vi "Version_4.9_8_on-chip_valves_for25ulSyringe_withModfied_Plunging.vi"() -> ()   [LabVIEW 2020] (continued)
                                n5068 = call "ProcessCompletionWaiter (SubVI).vi"("VISA Refnum in"=w5469) -> ()  [unwired: 11 in]
                                }
                                frame #2 {
                                # "Switch to Port-10"
                                # "Port-10 of the pump is conncted to column-2 of chip"
                                n5069 = local read "VISA Refnum in\nfor Pump"() -> (w5472:refnum<visa-resource-name>)
                                n5070 = call "PortChanger (SubVI).vi"("Port Number"="10", "VISA Refnum in"=w5472) -> ()  [unwired: 10 in]
                                }
                                frame #3 {
                                n5071 = local read "Stopper that ends \nthe main loops"() -> (w5473:bool)
                                n5072 = local read "VISA Refnum in\nfor Pump"() -> (w5474:refnum<visa-resource-name>)
                                n5073 = case shown="True" w5473 {
                                frame False {
                                }
                                frame True {
                                n5074 = local read "VISA Refnum in\nfor Pump"() -> (w5475:refnum<visa-resource-name>)
                                n5075 = call "HardStopCurrentProcess (SubVI).vi"("VISA Refnum in"=w5475) -> ()  [unwired: 11 in]
                                }
                                }
                                n5076 = call "ProcessCompletionWaiter (SubVI).vi"("VISA Refnum in"=w5474) -> ()  [unwired: 11 in]
                                }
                                frame #4 {
                                # "Keeps the AMF valve after column-1 open and valve after column-2 closed"
                                n5077 = local read "Buffer-A2 Pumping\nResolution"() -> (w5487:T2)
                                n5078 = local read "VISA Refnum in\nfor Pump"() -> (w5489:refnum<visa-resource-name>)
                                n5079 = local read "f"() -> (w5481:dbl)
                                n5080 = local write "Valve V3 Open"(TRUE ("Valve V3 Open")) -> ()
                                n5081 = local write "Valve V2 Open"(FALSE ("Valve V2 Open")) -> ()
                                n5082 = local write "Valve V4 Open"(TRUE ("Valve V4 Open")) -> ()
                                n5083 = local write "Valve V1 Open"(FALSE ("Valve V1 Open")) -> ()
                                n5084 = local read "Volume of Syringe"() -> (w5488:dbl)
                                n5085 = call "GoToAbsolutePosition(SubVI).vi"("Absolute Volume Position in Syringe (in ul)"=0.0 ("Volume to be Dispensed"), "Volume of Syringe"=w5488, "Resolution of Pumping"=w5487, "Flow Rate (ul/min)"=w5481, "VISA Refnum in"=w5489) -> ()  [unwired: 6 in, 1 out]
                                n5086 = local write "External Valve \nOpen"(FALSE ("External Valve \nOpen")) -> ()
                                n5087 = local write "Valve V8 Open"(FALSE ("Valve V8 Open")) -> ()
                                n5088 = local write "Valve V5 Open"(TRUE ("Valve V5 Open")) -> ()
                                n5089 = local write "Valve V6 Open"(FALSE ("Valve V6 Open")) -> ()
                                n5090 = local write "Valve V7 Open"(TRUE ("Valve V7 Open")) -> ()
                                }
                                frame #5 {
                                n5091 = local read "VISA Refnum in\nfor Pump"() -> (w5490:refnum<visa-resource-name>)
                                n5092 = call "ProcessCompletionWaiter (SubVI).vi"("VISA Refnum in"=w5490) -> ()  [unwired: 11 in]
                                }
                                frame #6 {
                                # "Change the port back to Buffer-C1"
                                n5093 = local read "VISA Refnum in\nfor Pump"() -> (w5492:refnum<visa-resource-name>)
                                n5094 = local read "Port for \nC1-Equilibriation"() -> (w5491:string)
                                n5095 = call "PortChanger (SubVI).vi"("Port Number"=w5491, "VISA Refnum in"=w5492) -> ()  [unwired: 10 in]
                                }
                                frame #7 {
                                n5096 = local read "VISA Refnum in\nfor Pump"() -> (w5493:refnum<visa-resource-name>)
                                n5097 = call "ProcessCompletionWaiter (SubVI).vi"("VISA Refnum in"=w5493) -> ()  [unwired: 11 in]
                                }
                              }
                            }
                            n5098 = local write "Reminder of the \nVolume to be \nPumped"(w5460) -> ()
                          }
                          frame #5 {
                            # "Washes the SEC column"
                            n5099 = stacked-sequence {
                              frame #0 {
                                n5100 = local read "Buffer-A2 Pumping\nResolution"() -> (w5496:T2)
                                n5101 = local read "VISA Refnum in\nfor Pump"() -> (w5498:refnum<visa-resource-name>)
                                n5102 = local read "Reminder of the \nVolume to be \nPumped"() -> (w5494:dbl)
                                n5103 = local read "Volume of Syringe"() -> (w5497:dbl)
                                n5104 = call "RPickUp(SubVI).vi"("Volume to be picked up"=w5494, "Volume of Syringe"=w5497, "Resolution of PickUP"=w5496, "PickUp Flow Rate (ul/min)"=150.0, "VISA Refnum in"=w5498) -> ()  [unwired: 6 in, 1 out]
                              }
                              frame #1 {
                                n5105 = local read "Stopper that ends \nthe main loops"() -> (w5499:bool)
                                n5106 = local read "VISA Refnum in\nfor Pump"() -> (w5500:refnum<visa-resource-name>)
                                n5107 = case shown="True" w5499 {
                                frame False {
                                }
                                frame True {
                                n5108 = local read "VISA Refnum in\nfor Pump"() -> (w5501:refnum<visa-resource-name>)
                                n5109 = call "HardStopCurrentProcess (SubVI).vi"("VISA Refnum in"=w5501) -> ()  [unwired: 11 in]
                                }
                                }
                                n5110 = call "ProcessCompletionWaiter (SubVI).vi"("VISA Refnum in"=w5500) -> ()  [unwired: 11 in]
                              }
                              frame #2 {
                                # "Switch to Port-10"
                                # "Port-10 of the pump is conncted to column-2 of chip"
                                n5111 = local read "VISA Refnum in\nfor Pump"() -> (w5503:refnum<visa-resource-name>)
                                n5112 = call "PortChanger (SubVI).vi"("Port Number"="10", "VISA Refnum in"=w5503) -> ()  [unwired: 10 in]
                              }
                              frame #3 {
                                n5113 = local read "Stopper that ends \nthe main loops"() -> (w5504:bool)
                                n5114 = local read "VISA Refnum in\nfor Pump"() -> (w5505:refnum<visa-resource-name>)
                                n5115 = case shown="True" w5504 {
                                frame False {
                                }
                                frame True {
                                n5116 = local read "VISA Refnum in\nfor Pump"() -> (w5506:refnum<visa-resource-name>)
                                n5117 = call "HardStopCurrentProcess (SubVI).vi"("VISA Refnum in"=w5506) -> ()  [unwired: 11 in]
                                }
                                }
                                n5118 = call "ProcessCompletionWaiter (SubVI).vi"("VISA Refnum in"=w5505) -> ()  [unwired: 11 in]
                              }
                              frame #4 {
                                n5119 = local read "Buffer-A2 Pumping\nResolution"() -> (w5518:T2)
                                n5120 = local read "VISA Refnum in\nfor Pump"() -> (w5520:refnum<visa-resource-name>)
                                n5121 = local read "f"() -> (w5512:dbl)
                                n5122 = local read "Volume of Syringe"() -> (w5519:dbl)
                                n5123 = call "GoToAbsolutePosition(SubVI).vi"("Absolute Volume Position in Syringe (in ul)"=0.0 ("Volume to be Dispensed"), "Volume of Syringe"=w5519, "Resolution of Pumping"=w5518, "Flow Rate (ul/min)"=w5512, "VISA Refnum in"=w5520) -> ()  [unwired: 6 in, 1 out]
                                n5124 = local write "Valve V3 Open"(TRUE ("Valve V3 Open")) -> ()
                                n5125 = local write "Valve V2 Open"(FALSE ("Valve V2 Open")) -> ()
                                n5126 = local write "Valve V1 Open"(FALSE ("Valve V1 Open")) -> ()
                                n5127 = local write "Valve V4 Open"(TRUE ("Valve V4 Open")) -> ()
                                n5128 = local write "External Valve \nOpen"(FALSE ("External Valve \nOpen")) -> ()
                                n5129 = local write "Valve V8 Open"(FALSE ("Valve V8 Open")) -> ()
                                n5130 = local write "Valve V6 Open"(TRUE ("Valve V6 Open")) -> ()
                                n5131 = local write "Valve V5 Open"(TRUE ("Valve V5 Open")) -> ()
                                n5132 = local write "Valve V7 Open"(TRUE ("Valve V7 Open")) -> ()
                              }
                              frame #5 {
                                n5133 = local read "VISA Refnum in\nfor Pump"() -> (w5521:refnum<visa-resource-name>)
                                n5134 = call "ProcessCompletionWaiter (SubVI).vi"("VISA Refnum in"=w5521) -> ()  [unwired: 11 in]
                              }
                            }
                          }
                        }
                        n5135 = local write "Washing Column-2"(TRUE ("Washing Column-2")) -> ()
                      }
                      frame #4 {
                        # "Elute Column-1, Divert Sample into Column-2, Elute column-2 and Divert the sample onto Grid"
                        n5136 = stacked-sequence {
                          frame #0 {
                            # "Switch to Port-7"
                            # "Port-7 of pump is connected to Buffer-B"
                            n5137 = local write "Washing Column-2"(FALSE ("Washing Column-2")) -> ()
                            n5138 = local read "VISA Refnum in\nfor Pump"() -> (w5526:refnum<visa-resource-name>)
                            n5139 = local read "Port for \nB-Elution"() -> (w5524:string)
                            n5140 = local write "Affinity Elution On"(TRUE ("Affinity Elution On")) -> ()
                            n5141 = call "PortChanger (SubVI).vi"("Port Number"=w5524, "VISA Refnum in"=w5526) -> ()  [unwired: 10 in]
                            n5142 = local write "Elution of Column-1"(TRUE ("Elution of Column-1")) -> ()
                          }
                          frame #1 {
                            n5143 = local read "VISA Refnum in\nfor Pump"() -> (w5527:refnum<visa-resource-name>)
                            n5144 = call "ProcessCompletionWaiter (SubVI).vi"("VISA Refnum in"=w5527) -> ()  [unwired: 11 in]
                          }
                          frame #2 {
                            # "If Yes, it will clean the elution buffer from port-5 tubing a bit more"
                            n5145 = stacked-sequence {
                              frame #0 {
                                n5146 = local read "Buffer-B Pumping\nResolution"() -> (w5530:T2)
                                n5147 = local read "VISA Refnum in\nfor Pump"() -> (w5532:refnum<visa-resource-name>)
                                n5148 = local read "V-S"() -> (w5529:dbl)
                                n5149 = local read "Volume of Syringe"() -> (w5531:dbl)
                                n5150 = call "RPickUp(SubVI).vi"("Volume to be picked up"=w5529, "Volume of Syringe"=w5531, "Resolution of PickUP"=w5530, "PickUp Flow Rate (ul/min)"=150.0, "VISA Refnum in"=w5532) -> ()  [unwired: 6 in, 1 out]
                              }
                              frame #1 {
                                n5151 = local read "Stopper that ends \nthe main loops"() -> (w5533:bool)
                                n5152 = local read "VISA Refnum in\nfor Pump"() -> (w5534:refnum<visa-resource-name>)
                                n5153 = case shown="True" w5533 {
                                frame False {
                                }
                                frame True {
                                n5154 = local read "VISA Refnum in\nfor Pump"() -> (w5535:refnum<visa-resource-name>)
                                n5155 = call "HardStopCurrentProcess (SubVI).vi"("VISA Refnum in"=w5535) -> ()  [unwired: 11 in]
                                }
                                }
                                n5156 = call "ProcessCompletionWaiter (SubVI).vi"("VISA Refnum in"=w5534) -> ()  [unwired: 11 in]
                              }
                              frame #2 {
                                n5157 = local read "VISA Refnum in\nfor Pump"() -> (w5537:refnum<visa-resource-name>)
                                n5158 = call "PortChanger (SubVI).vi"("Port Number"="1", "VISA Refnum in"=w5537) -> ()  [unwired: 10 in]
                              }
                              frame #3 {
                                n5159 = local read "Stopper that ends \nthe main loops"() -> (w5538:bool)
                                n5160 = local read "VISA Refnum in\nfor Pump"() -> (w5539:refnum<visa-resource-name>)
                                n5161 = case shown="True" w5538 {
                                frame False {
                                }
                                frame True {
                                n5162 = local read "VISA Refnum in\nfor Pump"() -> (w5540:refnum<visa-resource-name>)
                                n5163 = call "HardStopCurrentProcess (SubVI).vi"("VISA Refnum in"=w5540) -> ()  [unwired: 11 in]
                                }
                                }
                                n5164 = call "ProcessCompletionWaiter (SubVI).vi"("VISA Refnum in"=w5539) -> ()  [unwired: 11 in]
                              }
                              frame #4 {
                                n5165 = local read "VISA Refnum in\nfor Pump"() -> (w5545:refnum<visa-resource-name>)
                                n5166 = local read "Volume of Syringe"() -> (w5542:dbl)
                                n5167 = call "GoToAbsolutePosition(SubVI).vi"("Absolute Volume Position in Syringe (in ul)"=0.0, "Volume of Syringe"=w5542, "Resolution of Pumping"=T2."Standard Pumping", "Flow Rate (ul/min)"=150.0, "VISA Refnum in"=w5545) -> ()  [unwired: 6 in, 1 out]
                              }
                              frame #5 {
                                n5168 = local read "Stopper that ends \nthe main loops"() -> (w5546:bool)
                                n5169 = local read "VISA Refnum in\nfor Pump"() -> (w5547:refnum<visa-resource-name>)
                                n5170 = case shown="True" w5546 {
                                frame False {
                                }
                                frame True {
                                n5171 = local read "VISA Refnum in\nfor Pump"() -> (w5548:refnum<visa-resource-name>)
                                n5172 = call "HardStopCurrentProcess (SubVI).vi"("VISA Refnum in"=w5548) -> ()  [unwired: 11 in]
                                }
                                }
                                n5173 = call "ProcessCompletionWaiter (SubVI).vi"("VISA Refnum in"=w5547) -> ()  [unwired: 11 in]
                              }
                            }
                          }
                          frame #3 {
                            n5174 = local read "VISA Refnum in\nfor Pump"() -> (w5550:refnum<visa-resource-name>)
                            n5175 = local read "Port for \nB-Elution"() -> (w5549:string)
                            n5176 = call "PortChanger (SubVI).vi"("Port Number"=w5549, "VISA Refnum in"=w5550) -> ()  [unwired: 10 in]
                          }
                          frame #4 {
                            n5177 = local read "VISA Refnum in\nfor Pump"() -> (w5551:refnum<visa-resource-name>)
                            n5178 = call "ProcessCompletionWaiter (SubVI).vi"("VISA Refnum in"=w5551) -> ()  [unwired: 11 in]
                          }
                          frame #5 {
                            n5179 = local read "Buffer-B PickUp \nFlow Rate (ul/min)"() -> (w5554:dbl)
                            n5180 = local read "Buffer-B Pumping\nResolution"() -> (w5553:T2)
                            n5181 = local read "VISA Refnum in\nfor Pump"() -> (w5556:refnum<visa-resource-name>)
                            n5182 = local read "Buffer-B Volume \nto be  Pumped"() -> (w5552:dbl)
                            n5183 = local read "Volume of Syringe"() -> (w5555:dbl)
                            n5184 = call "RPickUp(SubVI).vi"("Volume to be picked up"=w5552, "Volume of Syringe"=w5555, "Resolution of PickUP"=w5553, "PickUp Flow Rate (ul/min)"=w5554, "VISA Refnum in"=w5556) -> ()  [unwired: 6 in, 1 out]
                          }
                          frame #6 {
                            n5185 = local read "Stopper that ends \nthe main loops"() -> (w5557:bool)
                            n5186 = local read "VISA Refnum in\nfor Pump"() -> (w5558:refnum<visa-resource-name>)
                            n5187 = case shown="True" w5557 {
                              frame False {
                              }
                              frame True {
                                n5188 = local read "VISA Refnum in\nfor Pump"() -> (w5559:refnum<visa-resource-name>)
                                n5189 = call "HardStopCurrentProcess (SubVI).vi"("VISA Refnum in"=w5559) -> ()  [unwired: 11 in]
                              }
                            }
                            n5190 = call "ProcessCompletionWaiter (SubVI).vi"("VISA Refnum in"=w5558) -> ()  [unwired: 11 in]
                          }
                          frame #7 {
                            # "Reads the initial Plunger Position for computing the volume dispensed"
                            n5191 = local read "VISA Refnum in\nfor Pump"() -> (w5561:refnum<visa-resource-name>)
                            n5192 = call "AbsolutePlungerPosition (SubVI).vi"("VISA Refnum in"=w5561) -> ("Plunger Position"=w5560:i32)  [unwired: 10 in]
                            n5193 = local write "Initial Plunger Position"(w5560) -> ()
                          }
                          frame #8 {
                            # "Switch to Port-8"
                            # "Port-8 of the pump is conncted to elution port of column-1 of chip"
                            n5194 = local read "VISA Refnum in\nfor Pump"() -> (w5563:refnum<visa-resource-name>)
                            n5195 = call "PortChanger (SubVI).vi"("Port Number"="8", "VISA Refnum in"=w5563) -> ()  [unwired: 10 in]
                          }
                          frame #9 {
                            n5196 = local read "Stopper that ends \nthe main loops"() -> (w5564:bool)
                            n5197 = local read "VISA Refnum in\nfor Pump"() -> (w5565:refnum<visa-resource-name>)
                            n5198 = call "ProcessCompletionWaiter (SubVI).vi"("VISA Refnum in"=w5565) -> ()  [unwired: 11 in]
                            n5199 = case shown="True" w5564 {
                              frame False {
                              }
                              frame True {
                                n5200 = local read "VISA Refnum in\nfor Pump"() -> (w5566:refnum<visa-resource-name>)
                                n5201 = call "HardStopCurrentProcess (SubVI).vi"("VISA Refnum in"=w5566) -> ()  [unwired: 11 in]
                              }
                            }
                          }
                          frame #10 {
                            # "Discard first few microlitres of elution buffer"
                            # "Keeps the AMF valve after column-1 open and valve after column-2 closed"
                            n5202 = local write "Valve V1 Open"(FALSE ("Valve V1 Open")) -> ()
                            n5203 = local write "Valve V2 Open"(FALSE ("Valve V2 Open")) -> ()
                            n5204 = local write "Valve V3 Open"(FALSE ("Valve V3 Open")) -> ()
                            n5205 = local write "Valve V4 Open"(FALSE ("Valve V4 Open")) -> ()
                            n5206 = local write "External Valve \nOpen"(FALSE ("External Valve \nOpen")) -> ()
                            n5207 = local write "Valve V8 Open"(TRUE ("Valve V8 Open")) -> ()
                            n5208 = local write "Valve V6 Open"(FALSE ("Valve V6 Open")) -> ()
                            n5209 = local write "Valve V5 Open"(FALSE ("Valve V5 Open")) -> ()
                            n5210 = local write "Valve V7 Open"(FALSE ("Valve V7 Open")) -> ()
                          }
                          frame #11 {
                            n5211 = local read "Buffer-B Dispense\nFlow Rate (ul/min)"() -> (w5581:dbl)
                            n5212 = local read "Buffer-B Pumping\nResolution"() -> (w5580:T2)
                            n5213 = local read "Initial Plunger Position"() -> (w5577:dbl)
                            n5214 = local read "VISA Refnum in\nfor Pump"() -> (w5583:refnum<visa-resource-name>)
                            n5215 = local read "Volume of Syringe"() -> (w5582:dbl)
                            n5216 = call "GoToAbsolutePosition(SubVI).vi"("Absolute Volume Position in Syringe (in ul)"=0.0 ("Volume to be Dispensed"), "Volume of Syringe"=w5582, "Resolution of Pumping"=w5580, "Flow Rate (ul/min)"=w5581, "VISA Refnum in"=w5583) -> ()  [unwired: 6 in, 1 out]
                            n5217 = local write "Pause Data Collection"(FALSE ("Pause Data Collection")) -> ()
                            n5218 = local write "Vol_now"(0.0 ("Vol_now")) -> ()
                            n5219 = local write "Position\nNow"(w5577) -> ()
                          }
                          frame #12 {
                            n5220 = local read "Buffer-B Pumping\nResolution"() -> (w5588:T2)
                            n5221 = local read "VISA Refnum in\nfor Pump"() -> (w5589:refnum<visa-resource-name>)
                            n5222 = local read "Volume of Syringe"() -> (w5587:dbl)
                            n5223 = local read "Position\nNow"() -> (w5584:dbl)
                            n5224 = local read "Pause Elution"() -> (w5585:bool)
                            n5225 = case shown="False" w5585 {
                              tunnel: w5584 -> [w5593 _]
                              tunnel: w5589 -> [w5592 w5634]
                              tunnel: w5588 -> [w5591 _]
                              tunnel: w5587 -> [w5590 _]
                              frame False {
                                n5226 = stacked-sequence {
                                tunnel: w5593 -> [_ w5599]
                                tunnel: w5592 -> [_ w5598]
                                tunnel: w5591 -> [_ w5597]
                                tunnel: w5590 -> [_ w5596]
                                frame #0 {
                                n5227 = Wait (ms)(milliseconds to wait=u32 3000) -> ()  [unwired: 1 out]
                                n5228 = local write "Signal"(TRUE ("Signal")) -> ()
                                }
                                frame #1 {
                                n5229 = while {
                                tunnel: w5599 -> [w5610]
                                tunnel: w5598 -> [w5609]
                                tunnel: w5597 -> [w5608]
                                tunnel: w5596 -> [w5607]
                                stop <- w5603 stop-if-true
                                n5230 = stacked-sequence {
                                tunnel: w5610 -> [_ w5617]
                                tunnel: w5609 -> [_ w5616]
                                tunnel: w5608 -> [_ w5615]
                                tunnel: w5607 -> [_ w5614]
                                frame #0 {
                                n5231 = Wait (ms)(milliseconds to wait=u32 500) -> ()  [unwired: 1 out]
                                }
                                frame #1 {
                                n5232 = call "AbsolutePlungerPosition (SubVI).vi"("VISA Refnum in"=w5616) -> ("Plunger Position"=w5613:i32)  [unwired: 10 in]
                                n5233 = case shown="\"High Resolution Pumping\"" w5615 {
                                tunnel: w5617 -> [w5622 w5631]
                                tunnel: w5613 -> [w5623 w5630]
                                tunnel: [w5621 w5628] -> w5612
                                tunnel: w5614 -> [w5620 w5629]
                                frame "Standard Pumping", Default {
                                n5234 = Subtract(x=w5622, y=w5623) -> (x-y=w5619:dbl)
                                n5235 = Absolute Value(x=w5619) -> (abs(x)=w5618:dbl)
                                n5236 = Multiply(x=w5618, y=w5620) -> (x*y=w5625:dbl)
                                n5237 = Divide(x=w5625, y=3000.0) -> (x/y=w5621:dbl)
                                }
                                frame "High Resolution Pumping" {
                                n5238 = Subtract(x=w5631, y=w5630) -> (x-y=w5627:dbl)
                                n5239 = Absolute Value(x=w5627) -> (abs(x)=w5626:dbl)
                                n5240 = Multiply(x=w5626, y=w5629) -> (x*y=w5633:dbl)
                                n5241 = Divide(x=w5633, y=24000.0) -> (x/y=w5628:dbl)
                                }
                                }
                                n5242 = local write "Volume being Injected \nin this process"(w5612) -> ()
                                }
                                }
                                n5243 = local read "Volume being Injected \nin this process"() -> (w5601:dbl)
                                n5244 = local read "Discard volume \npriot to elution"() -> (w5602:dbl)
                                n5245 = local read "Divert Elution Buffer\ninto Column-1"() -> (w5606:bool)
                                n5246 = local read "Stopper that ends \nthe main loops"() -> (w5605:bool)
                                n5247 = Greater Or Equal?(x=w5601, y=w5602) -> (x >= y?=w5600:bool)
                                n5248 = Or(x=w5606, y=w5605) -> (x .or. y?=w5604:bool)
                                n5249 = Or(x=w5600, y=w5604) -> (x .or. y?=w5603:bool)
                                }
                                }
                                }
                              }
                              frame True {
                                n5250 = stacked-sequence {
                                tunnel: w5634 -> [_ w5637 _]
                                frame #0 {
                                n5251 = Wait (ms)(milliseconds to wait=u32 2000) -> ()  [unwired: 1 out]
                                }
                                frame #1 {
                                n5252 = local read "Signal"() -> (w5636:bool)
                                n5253 = case shown="True" w5636 {
                                tunnel: w5637 -> [_ w5643]
                                frame False {
                                }
                                frame True {
                                n5254 = local read "Volume being Injected \nin this process"() -> (w5641:dbl)
                                n5255 = local read "Net Elution \nVolume"() -> (w5640:dbl)
                                n5256 = local write "Signal"(FALSE ("Signal")) -> ()
                                n5257 = Add(x=w5641, y=w5640) -> (x+y=w5639:dbl)
                                n5258 = call "AbsolutePlungerPosition (SubVI).vi"("VISA Refnum in"=w5643) -> ("Plunger Position"=w5642:i32)  [unwired: 10 in]
                                n5259 = local write "Net Elution \nVolume"(w5639) -> ()
                                n5260 = local write "Position\nNow"(w5642) -> ()
                                }
                                }
                                }
                                frame #2 {
                                n5261 = local write "Volume being Injected \nin this process"(0.0 ("Volume being Injected \nin this process")) -> ()
                                }
                                }
                              }
                            }
                            n5262 = local read "Stopper that ends \nthe main loops"() -> (w5586:bool)
                            n5263 = case shown="True" w5586 {
                              frame False {
                              }
                              frame True {
                                n5264 = local read "VISA Refnum in\nfor Pump"() -> (w5645:refnum<visa-resource-name>)
                                n5265 = call "HardStopCurrentProcess (SubVI).vi"("VISA Refnum in"=w5645) -> ()  [unwired: 11 in]
                              }
                            }
                          }
                          frame #13 {
                            # "Keeps the AMF valve after column-1 open and valve after column-2 closed"
                            n5266 = local write "Valve V1 Open"(TRUE ("Valve V1 Open")) -> ()
                            n5267 = local write "Valve V2 Open"(TRUE ("Valve V2 Open")) -> ()
                            n5268 = local write "Valve V3 Open"(FALSE ("Valve V3 Open")) -> ()
                            n5269 = local write "Valve V4 Open"(FALSE ("Valve V4 Open")) -> ()
                            n5270 = local write "External Valve \nOpen"(TRUE ("External Valve \nOpen")) -> ()
                            n5271 = local write "Valve V8 Open"(FALSE ("Valve V8 Open")) -> ()
                            n5272 = local write "Valve V6 Open"(FALSE ("Valve V6 Open")) -> ()
                            n5273 = local write "Valve V5 Open"(FALSE ("Valve V5 Open")) -> ()
                            n5274 = local write "Valve V7 Open"(FALSE ("Valve V7 Open")) -> ()
                          }
                          frame #14 {
                            n5275 = while {
                              stop <- w5661 stop-if-true
                              n5276 = event shown="[1] \"Divert Sample  into Column-2\": Value Change" {
                                selector: _ -> [_ _ _ _]
                                dyn-events: _ -> [_ _ _ _]
                                timeout: 100 -> [_ _ _ _]
                                tunnel: [_ _ w5676 _] -> w5660
                                tunnel: [_ w5675 _ _] -> w5659
                                event "Pause Elution\nValue": Value Change {
                                n5277 = event-data() -> ()  [unwired: 1 in, 6 out]
                                n5278 = stacked-sequence {
                                frame #0 {
                                n5279 = local read "Pause Elution"() -> (w5663:bool)
                                n5280 = case shown="False" w5663 {
                                frame False {
                                n5281 = local write "Pause Elution"(TRUE ("Pause Elution")) -> ()
                                }
                                frame True {
                                n5282 = local write "Pause Elution"(FALSE ("Pause Elution")) -> ()
                                }
                                }
                                }
                                frame #1 {
                                n5283 = local read "Pause Elution"() -> (w5666:bool)
                                n5284 = case shown="False" w5666 {
                                frame False {
                                n5285 = local read "Buffer-B Dispense\nFlow Rate (ul/min)"() -> (w5671:dbl)
                                n5286 = local read "VISA Refnum in\nfor Pump"() -> (w5672:refnum<visa-resource-name>)
                                n5287 = local read "Buffer-B Pumping\nResolution"() -> (w5668:T2)
                                n5288 = local read "Volume of Syringe"() -> (w5669:dbl)
                                n5289 = call "GoToAbsolutePosition(SubVI).vi"("Absolute Volume Position in Syringe (in ul)"=0.0, "Volume of Syringe"=w5669, "Resolution of Pumping"=w5668, "Flow Rate (ul/min)"=w5671, "VISA Refnum in"=w5672) -> ()  [unwired: 6 in, 1 out]
                                n5290 = local write "Pause Data Collection"(FALSE ("Pause Data Collection")) -> ()
                                }
                                frame True {
                                n5291 = local read "VISA Refnum in\nfor Pump"() -> (w5674:refnum<visa-resource-name>)
                                n5292 = local write "Pause Data Collection"(TRUE ("Pause Data Collection")) -> ()
                                n5293 = call "HardStopCurrentProcess (SubVI).vi"("VISA Refnum in"=w5674) -> ()  [unwired: 11 in]
                                }
                                }
                                }
                                }
                                }
                                event "Divert Sample \ninto Column-2": Value Change {
                                n5294 = event-data() -> ()  [unwired: 1 in, 6 out]
                                n5295 = local read "Divert Sample \ninto Column-2"() -> (w5675:bool)
                                }
                                event "Stop for End of \nExperiment \nand Data Writing": Value Change {
                                n5296 = event-data() -> ()  [unwired: 1 in, 6 out]
                                n5297 = local read "Stop for End of \nExperiment \nand Data Writing"() -> (w5676:bool)
                                }
                                event Timeout {
                                n5298 = event-data() -> ()  [unwired: 1 in, 3 out]
                                }
                              }
                              n5299 = Or(x=w5659, y=w5660) -> (x .or. y?=w5661:bool)
                            }
                            n5300 = local read "Buffer-B Pumping\nResolution"() -> (w5657:T2)
                            n5301 = local read "VISA Refnum in\nfor Pump"() -> (w5658:refnum<visa-resource-name>)
                            n5302 = local read "Volume of Syringe"() -> (w5656:dbl)
                            n5303 = while {
                              tunnel: w5658 -> [w5685]
                              tunnel: w5657 -> [w5684]
                              tunnel: w5656 -> [w5683]
                              stop <- w5679 stop-if-true
                              n5304 = local read "Position\nNow"() -> (w5677:dbl)
                              n5305 = local read "Pause Elution"() -> (w5678:bool)
                              n5306 = case shown="False" w5678 {
                                tunnel: w5677 -> [w5689 _]
                                tunnel: w5685 -> [w5688 w5731]
                                tunnel: w5684 -> [w5687 _]
                                tunnel: w5683 -> [w5686 _]
                                frame False {
                                n5307 = stacked-sequence {
                                tunnel: w5689 -> [_ w5695]
                                tunnel: w5688 -> [_ w5694]
                                tunnel: w5687 -> [_ w5693]
                                tunnel: w5686 -> [_ w5692]
                                frame #0 {
                                n5308 = Wait (ms)(milliseconds to wait=u32 3000) -> ()  [unwired: 1 out]
                                n5309 = local write "Signal"(TRUE ("Signal")) -> ()
                                }
                                frame #1 {
                                n5310 = while {
                                tunnel: w5695 -> [w5707]
                                tunnel: w5694 -> [w5706]
                                tunnel: w5693 -> [w5705]
                                tunnel: w5692 -> [w5704]
                                stop <- w5699 stop-if-true
                                n5311 = stacked-sequence {
                                tunnel: w5707 -> [_ w5714]
                                tunnel: w5706 -> [_ w5713]
                                tunnel: w5705 -> [_ w5712]
                                tunnel: w5704 -> [_ w5711]
                                frame #0 {
                                n5312 = Wait (ms)(milliseconds to wait=u32 500) -> ()  [unwired: 1 out]
                                }
                                frame #1 {
                                n5313 = call "AbsolutePlungerPosition (SubVI).vi"("VISA Refnum in"=w5713) -> ("Plunger Position"=w5710:i32)  [unwired: 10 in]
                                n5314 = case shown="\"High Resolution Pumping\"" w5712 {
                                tunnel: w5714 -> [w5719 w5728]
                                tunnel: w5710 -> [w5720 w5727]
                                tunnel: [w5718 w5725] -> w5709
                                tunnel: w5711 -> [w5717 w5726]
                                frame "Standard Pumping", Default {
                                n5315 = Subtract(x=w5719, y=w5720) -> (x-y=w5716:dbl)
                                n5316 = Absolute Value(x=w5716) -> (abs(x)=w5715:dbl)
                                n5317 = Multiply(x=w5715, y=w5717) -> (x*y=w5722:dbl)
                                n5318 = Divide(x=w5722, y=3000.0) -> (x/y=w5718:dbl)
                                }
                                frame "High Resolution Pumping" {
                                n5319 = Subtract(x=w5728, y=w5727) -> (x-y=w5724:dbl)
                                n5320 = Absolute Value(x=w5724) -> (abs(x)=w5723:dbl)
                                n5321 = Multiply(x=w5723, y=w5726) -> (x*y=w5730:dbl)
                                n5322 = Divide(x=w5730, y=24000.0) -> (x/y=w5725:dbl)
                                }
                                }
                                n5323 = local write "Volume being Injected \nin this process"(w5709) -> ()
                                }
                                }
                                n5324 = local read "Volume being Injected \nin this process"() -> (w5697:dbl)
                                n5325 = local read "Affinity Elution \nGraph Min CutOff"() -> (w5696:dbl)
                                n5326 = local read "Stopper that ends \nthe main loops"() -> (w5702:bool)
                                n5327 = local read "Divert Sample \ninto Column-2"() -> (w5703:bool)
                                n5328 = Greater Or Equal?(x=w5697, y=w5696) -> (x >= y?=w5698:bool)
                                n5329 = Or(x=w5703, y=w5702) -> (x .or. y?=w5700:bool)
                                n5330 = local read "Pause Elution"() -> (w5701:bool)
                                n5331 = local write "Affinity Elution \nis Approaching"(w5698) -> ()
                                n5332 = Or(x=w5701, y=w5700) -> (x .or. y?=w5699:bool)
                                }
                                }
                                }
                                }
                                frame True {
                                n5333 = stacked-sequence {
                                tunnel: w5731 -> [_ w5734 _]
                                frame #0 {
                                n5334 = Wait (ms)(milliseconds to wait=u32 2000) -> ()  [unwired: 1 out]
                                }
                                frame #1 {
                                n5335 = local read "Signal"() -> (w5733:bool)
                                n5336 = case shown="True" w5733 {
                                tunnel: w5734 -> [_ w5740]
                                frame False {
                                }
                                frame True {
                                n5337 = local read "Volume being Injected \nin this process"() -> (w5738:dbl)
                                n5338 = local read "Net Elution \nVolume"() -> (w5737:dbl)
                                n5339 = local write "Signal"(FALSE ("Signal")) -> ()
                                n5340 = Add(x=w5738, y=w5737) -> (x+y=w5736:dbl)
                                n5341 = call "AbsolutePlungerPosition (SubVI).vi"("VISA Refnum in"=w5740) -> ("Plunger Position"=w5739:i32)  [unwired: 10 in]
                                n5342 = local write "Net Elution \nVolume"(w5736) -> ()
                                n5343 = local write "Position\nNow"(w5739) -> ()
                                }
                                }
                                }
                                frame #2 {
                                n5344 = local write "Volume being Injected \nin this process"(0.0 ("Volume being Injected \nin this process")) -> ()
                                }
                                }
                                }
                              }
                              n5345 = local read "Stopper that ends \nthe main loops"() -> (w5681:bool)
                              n5346 = local read "Divert Sample \ninto Column-2"() -> (w5680:bool)
                              n5347 = Or(x=w5680, y=w5681) -> (x .or. y?=w5679:bool)
                              n5348 = Wait (ms)(milliseconds to wait=u32 300) -> ()  [unwired: 1 out]
                            }
                            n5349 = local read "Stopper that ends \nthe main loops"() -> (w5655:bool)
                            n5350 = case shown="True" w5655 {
                              frame False {
                              }
                              frame True {
                                n5351 = local read "VISA Refnum in\nfor Pump"() -> (w5742:refnum<visa-resource-name>)
                                n5352 = call "HardStopCurrentProcess (SubVI).vi"("VISA Refnum in"=w5742) -> ()  [unwired: 11 in]
                              }
                            }
                          }
                          frame #15 {
                            # "Keeps the on-chip Valve V1 and V3 after column-2 open"
                            # "Keeps the AMF valve after column-1 closed and valve after column-2 open"
                            n5353 = local read "VISA Refnum in\nfor Pump"() -> (w5755:refnum<visa-resource-name>)
                            n5354 = local read "Volume being Injected \nin this process"() -> (w5752:dbl)
                            n5355 = local write "Sample Volume Diverted\ninto Column-2"(0.0 ("Sample Volume Diverted\ninto Column-2")) -> ()
                            n5356 = call "AbsolutePlungerPosition (SubVI).vi"("VISA Refnum in"=w5755) -> ("Plunger Position"=w5754:i32)  [unwired: 10 in]
                            n5357 = local write "Position\nNow"(w5754) -> ()
                            n5358 = local write "Vol_previous"(0.0 ("Vol_diff")) -> ()
                            n5359 = local write "Vol_now"(w5752) -> ()
                            n5360 = local write "Valve V1 Open"(TRUE ("Valve V1 Open")) -> ()
                            n5361 = local write "Valve V3 Open"(FALSE ("Valve V3 Open")) -> ()
                            n5362 = local write "Valve V2 Open"(FALSE ("Valve V2 Open")) -> ()
                            n5363 = local write "Valve V4 Open"(TRUE ("Valve V4 Open")) -> ()
                            n5364 = local write "External Valve \nOpen"(FALSE ("External Valve \nOpen")) -> ()
                            n5365 = local write "Valve V8 Open"(FALSE ("Valve V8 Open")) -> ()
                            n5366 = local write "Valve V5 Open"(TRUE ("Valve V5 Open")) -> ()
                            n5367 = local write "Valve V6 Open"(FALSE ("Valve V6 Open")) -> ()
                            n5368 = local write "Valve V7 Open"(TRUE ("Valve V7 Open")) -> ()
                          }
                          frame #16 {
                            n5369 = local read "Divert Sample \ninto Column-2"() -> (w5757:bool)
                            n5370 = case shown="True" w5757 {
                              frame False {
                                n5371 = stacked-sequence {
                                frame #0 {
                                n5372 = local read "Buffer-B Pumping\nResolution"() -> (w5760:T2)
                                n5373 = local read "VISA Refnum in\nfor Pump"() -> (w5762:refnum<visa-resource-name>)
                                n5374 = local read "Initial Plunger Position"() -> (w5761:dbl)
                                n5375 = local read "Volume of Syringe"() -> (w5759:dbl)
                                n5376 = while {
                                tunnel: w5761 -> [w5768]
                                tunnel: w5762 -> [w5767]
                                tunnel: w5760 -> [w5766]
                                tunnel: w5759 -> [w5765]
                                stop <- w5763 stop-if-true
                                n5377 = Wait (ms)(milliseconds to wait=u32 100) -> ()  [unwired: 1 out]
                                n5378 = stacked-sequence {
                                tunnel: w5768 -> [w5774 _]
                                tunnel: w5767 -> [w5773 w5794]
                                tunnel: w5766 -> [w5772 _]
                                tunnel: w5765 -> [w5771 _]
                                tunnel: [_ w5792] -> w5763
                                frame #0 {
                                n5379 = call "AbsolutePlungerPosition (SubVI).vi"("VISA Refnum in"=w5773) -> ("Plunger Position"=w5770:i32)  [unwired: 10 in]
                                n5380 = case shown="\"Standard Pumping\", Default" w5772 {
                                tunnel: w5774 -> [w5779 w5788]
                                tunnel: w5770 -> [w5780 w5787]
                                tunnel: [w5778 w5785] -> w5769
                                tunnel: w5771 -> [w5777 w5786]
                                frame "Standard Pumping", Default {
                                n5381 = Subtract(x=w5779, y=w5780) -> (x-y=w5776:dbl)
                                n5382 = Absolute Value(x=w5776) -> (abs(x)=w5775:dbl)
                                n5383 = Multiply(x=w5775, y=w5777) -> (x*y=w5782:dbl)
                                n5384 = Divide(x=w5782, y=3000.0) -> (x/y=w5778:dbl)
                                }
                                frame "High Resolution Pumping" {
                                n5385 = Subtract(x=w5788, y=w5787) -> (x-y=w5784:dbl)
                                n5386 = Absolute Value(x=w5784) -> (abs(x)=w5783:dbl)
                                n5387 = Multiply(x=w5783, y=w5786) -> (x*y=w5790:dbl)
                                n5388 = Divide(x=w5790, y=24000.0) -> (x/y=w5785:dbl)
                                }
                                }
                                n5389 = local write "Volume being Injected \nin this process"(w5769) -> ()
                                }
                                frame #1 {
                                n5390 = local read "Stopper that ends \nthe main loops"() -> (w5791:bool)
                                n5391 = call "LSPOneStatus (SubVI).vi"("VISA Refnum in"=w5794) -> ("read buffer"=w5796:string)  [unwired: 10 in]
                                n5392 = call <vilib>:"Trim Whitespace.vi"("string"=w5796) -> ("trimmed string"=w5795:string)  [unwired: 1 in]
                                n5393 = Equal?(x=w5795, y="/0`\u0003") -> (x = y?=w5793:bool)
                                n5394 = Or(x=w5793, y=w5791) -> (x .or. y?=w5792:bool)
                                }
                                }
                                }
                                n5395 = local read "Stopper that ends \nthe main loops"() -> (w5758:bool)
                                n5396 = case shown="True" w5758 {
                                frame False {
                                }
                                frame True {
                                n5397 = local read "VISA Refnum in\nfor Pump"() -> (w5798:refnum<visa-resource-name>)
                                n5398 = call "HardStopCurrentProcess (SubVI).vi"("VISA Refnum in"=w5798) -> ()  [unwired: 11 in]
                                }
                                }
                                }
                                }
                              }
                              frame True {
                                n5399 = stacked-sequence {
                                frame #0 {
                                n5400 = local read "Buffer-B Pumping\nResolution"() -> (w5801:T2)
                                n5401 = local read "VISA Refnum in\nfor Pump"() -> (w5803:refnum<visa-resource-name>)
                                n5402 = local read "Volume of Syringe"() -> (w5800:dbl)
                                n5403 = local read "Position\nNow"() -> (w5802:dbl)
                                n5404 = while {
                                tunnel: w5802 -> [w5809]
                                tunnel: w5803 -> [w5808]
                                tunnel: w5801 -> [w5807]
                                tunnel: w5800 -> [w5806]
                                stop <- w5804 stop-if-true
                                n5405 = Wait (ms)(milliseconds to wait=u32 100) -> ()  [unwired: 1 out]
                                n5406 = stacked-sequence {
                                tunnel: w5809 -> [w5819 _ _]
                                tunnel: w5808 -> [w5818 _ w5845]
                                tunnel: w5807 -> [w5817 _ _]
                                tunnel: w5806 -> [w5816 _ _]
                                tunnel: [_ _ w5843] -> w5804
                                frame #0 {
                                n5407 = local read "Vol_previous"() -> (w5813:dbl)
                                n5408 = call "AbsolutePlungerPosition (SubVI).vi"("VISA Refnum in"=w5818) -> ("Plunger Position"=w5815:i32)  [unwired: 10 in]
                                n5409 = case shown="\"Standard Pumping\", Default" w5817 {
                                tunnel: w5819 -> [w5824 w5833]
                                tunnel: w5815 -> [w5825 w5832]
                                tunnel: [w5823 w5830] -> w5814
                                tunnel: w5816 -> [w5822 w5831]
                                frame "Standard Pumping", Default {
                                n5410 = Subtract(x=w5824, y=w5825) -> (x-y=w5821:dbl)
                                n5411 = Absolute Value(x=w5821) -> (abs(x)=w5820:dbl)
                                n5412 = Multiply(x=w5820, y=w5822) -> (x*y=w5827:dbl)
                                n5413 = Divide(x=w5827, y=3000.0) -> (x/y=w5823:dbl)
                                }
                                frame "High Resolution Pumping" {
                                n5414 = Subtract(x=w5833, y=w5832) -> (x-y=w5829:dbl)
                                n5415 = Absolute Value(x=w5829) -> (abs(x)=w5828:dbl)
                                n5416 = Multiply(x=w5828, y=w5831) -> (x*y=w5835:dbl)
                                n5417 = Divide(x=w5835, y=24000.0) -> (x/y=w5830:dbl)
                                }
                                }
                                n5418 = Subtract(x=w5814, y=w5813) -> (x-y=w5812:dbl)
                                n5419 = local read "Vol_now"() -> (w5810:dbl)
                                n5420 = local write "Sample Volume Diverted\ninto Column-2"(w5814) -> ()
                                n5421 = Add(x=w5812, y=w5810) -> (x+y=w5811:dbl)
                                n5422 = local write "Volume being Injected \nin this process"(w5811) -> ()
                                }
                                frame #1 {
                                n5423 = local read "Volume being Injected \nin this process"() -> (w5836:dbl)
                                n5424 = local read "Sample Volume Diverted\ninto Column-2"() -> (w5837:dbl)
                                n5425 = local write "Vol_now"(w5836) -> ()
                                n5426 = local write "Vol_previous"(w5837) -> ()
                                }
                                frame #2 {
                                n5427 = local read "Buffer-B Volume \nto be Pumped for\nSample Diversion\nto Column-2"() -> (w5839:dbl)
                                n5428 = local read "Sample Volume Diverted\ninto Column-2"() -> (w5838:dbl)
                                n5429 = local read "Stopper that ends \nthe main loops"() -> (w5840:bool)
                                n5430 = call "LSPOneStatus (SubVI).vi"("VISA Refnum in"=w5845) -> ("read buffer"=w5847:string)  [unwired: 10 in]
                                n5431 = call <vilib>:"Trim Whitespace.vi"("string"=w5847) -> ("trimmed string"=w5846:string)  [unwired: 1 in]
                                n5432 = Equal?(x=w5846, y="/0`\u0003") -> (x = y?=w5844:bool)
                                n5433 = Greater Or Equal?(x=w5838, y=w5839) -> (x >= y?=w5842:bool)
                                n5434 = Or(x=w5840, y=w5842) -> (x .or. y?=w5841:bool)
                                n5435 = Or(x=w5844, y=w5841) -> (x .or. y?=w5843:bool)
                                }
                                }
                                }
                                n5436 = local read "Stopper that ends \nthe main loops"() -> (w5799:bool)
                                n5437 = case shown="True" w5799 {
                                frame False {
                                }
                                frame True {
                                n5438 = local read "VISA Refnum in\nfor Pump"() -> (w5849:refnum<visa-resource-name>)
                                n5439 = call "HardStopCurrentProcess (SubVI).vi"("VISA Refnum in"=w5849) -> ()  [unwired: 11 in]
                                }
                                }
                                }
                                frame #1 {
                                n5440 = local read "VISA Refnum in\nfor Pump"() -> (w5851:refnum<visa-resource-name>)
                                n5441 = local write "Pause Data Collection"(TRUE ("Pause Data Collection")) -> ()
                                n5442 = call "HardStopCurrentProcess (SubVI).vi"("VISA Refnum in"=w5851) -> ()  [unwired: 11 in]
                                }
                                frame #2 {
                                n5443 = local read "VISA Refnum in\nfor Pump"() -> (w5852:refnum<visa-resource-name>)
                                n5444 = call "PortChanger (SubVI).vi"("Port Number"="1", "VISA Refnum in"=w5852) -> ()  [unwired: 10 in]
                                }
                                frame #3 {
                                n5445 = local read "VISA Refnum in\nfor Pump"() -> (w5858:refnum<visa-resource-name>)
                                n5446 = local read "Volume of Syringe"() -> (w5854:dbl)
                                n5447 = call "GoToAbsolutePosition(SubVI).vi"("Absolute Volume Position in Syringe (in ul)"=0.0, "Volume of Syringe"=w5854, "Resolution of Pumping"=T2."Standard Pumping", "Flow Rate (ul/min)"=150.0, "VISA Refnum in"=w5858) -> ()  [unwired: 6 in, 1 out]
                                }
                                frame #4 {
                                n5448 = local read "VISA Refnum in\nfor Pump"() -> (w5860:refnum<visa-resource-name>)
                                n5449 = local write "Divert Sample \ninto Column-2"(FALSE ("Divert Sample \ninto Column-2")) -> ()
                                n5450 = call "ProcessCompletionWaiter (SubVI).vi"("VISA Refnum in"=w5860) -> ()  [unwired: 11 in]
                                }
                                }
                              }
                            }
                          }
                          frame #17 {
                            # "Keeps the On-Chip Valves V1 and V3 closed"
                            # "Switch to Port-5/8"
                            # "Port-5/8 of pump is connected to Buffer-C1/C2"
                            # "Keeps the AMF valve after column-1 open and valve after column-2 closed"
                            n5451 = local read "VISA Refnum in\nfor Pump"() -> (w5873:refnum<visa-resource-name>)
                            n5452 = local write "Pause Data Collection"(TRUE ("Pause Data Collection")) -> ()
                            n5453 = Wait (ms)(milliseconds to wait=u32 500) -> ()  [unwired: 1 out]
                            n5454 = local write "Affinity On"(FALSE ("Affinity On")) -> ()
                            n5455 = local read "Port for \nC2-Elution"() -> (w5866:string)
                            n5456 = local write "Affinity Elution On"(FALSE ("Affinity Elution On")) -> ()
                            n5457 = call "PortChanger (SubVI).vi"("Port Number"=w5866, "VISA Refnum in"=w5873) -> ()  [unwired: 10 in]
                            n5458 = local write "Valve V1 Open"(FALSE ("Valve V1 Open")) -> ()
                            n5459 = local write "Valve V2 Open"(FALSE ("Valve V2 Open")) -> ()
                            n5460 = local write "Valve V3 Open"(FALSE ("Valve V3 Open")) -> ()
                            n5461 = local write "Valve V4 Open"(FALSE ("Valve V4 Open")) -> ()
                            n5462 = local write "External Valve \nOpen"(FALSE ("External Valve \nOpen")) -> ()
                            n5463 = local write "Valve V8 Open"(FALSE ("Valve V8 Open")) -> ()
                            n5464 = local write "Valve V5 Open"(FALSE ("Valve V5 Open")) -> ()
                            n5465 = local write "Valve V6 Open"(FALSE ("Valve V6 Open")) -> ()
                            n5466 = local write "Valve V7 Open"(FALSE ("Valve V7 Open")) -> ()
                          }
                          frame #18 {
                            n5467 = local read "VISA Refnum in\nfor Pump"() -> (w5877:refnum<visa-resource-name>)
                            n5468 = call "ProcessCompletionWaiter (SubVI).vi"("VISA Refnum in"=w5877) -> ()  [unwired: 11 in]
                            n5469 = local write "Start the Process"(FALSE ("Start the Process")) -> ()
                          }
                          frame #19 {
                            n5470 = local read "Stopper that ends \nthe main loops"() -> (w5881:bool)
                            n5471 = local read "Start the Process"() -> (w5882:bool)
                            n5472 = Or(x=w5882, y=w5881) -> (x .or. y?=w5880:bool)
                            n5473 = local write "Elution of Column-1"(FALSE ("Elution of Column-1")) -> ()
                            n5474 = case shown="False" w5880 {
                              frame False {
                                n5475 = while {
                                stop <- w5886 stop-if-true
                                n5476 = local read "Stopper that ends \nthe main loops"() -> (w5887:bool)
                                n5477 = local read "Start the Process"() -> (w5888:bool)
                                n5478 = Or(x=w5888, y=w5887) -> (x .or. y?=w5886:bool)
                                n5479 = Wait (ms)(milliseconds to wait=u32 10) -> ()  [unwired: 1 out]
                                }
                                n5480 = One Button Dialog(message="Move to Column-2 detection zone and Press 'Start the Process' Button.") -> ()  [unwired: 1 in, 1 out]
                              }
                              frame True {
                              }
                            }
                            n5481 = local write "Volume being Injected \nin this process"(0.0 ("Volume being Injected \nin this process")) -> ()
                            n5482 = local write "Elution of Column-2"(TRUE ("Elution of Column-2")) -> ()
                          }
                          frame #20 {
                            # "If Yes, it will clean the SEC buffer from port-8 tubing else it will clean the pump valve a bit"
                            n5483 = local read "Clean the \nBuffer-C2 tubing"() -> (w5889:bool)
                            n5484 = case shown="False" w5889 {
                              frame False {
                                n5485 = stacked-sequence {
                                frame #0 {
                                n5486 = local read "VISA Refnum in\nfor Pump"() -> (w5891:refnum<visa-resource-name>)
                                n5487 = local read "Port for \nC2-Elution"() -> (w5890:string)
                                n5488 = call "PortChanger (SubVI).vi"("Port Number"=w5890, "VISA Refnum in"=w5891) -> ()  [unwired: 10 in]
                                }
                                frame #1 {
                                n5489 = local read "VISA Refnum in\nfor Pump"() -> (w5892:refnum<visa-resource-name>)
                                n5490 = call "ProcessCompletionWaiter (SubVI).vi"("VISA Refnum in"=w5892) -> ()  [unwired: 11 in]
                                }
                                frame #2 {
                                n5491 = local read "Buffer-C2 Pumping\nResolution"() -> (w5895:T2)
                                n5492 = local read "VISA Refnum in\nfor Pump"() -> (w5897:refnum<visa-resource-name>)
                                n5493 = local read "V-S"() -> (w5893:dbl)
                                n5494 = local read "Volume of Syringe"() -> (w5896:dbl)
                                n5495 = call "RPickUp(SubVI).vi"("Volume to be picked up"=w5893, "Volume of Syringe"=w5896, "Resolution of PickUP"=w5895, "PickUp Flow Rate (ul/min)"=150.0, "VISA Refnum in"=w5897) -> ()  [unwired: 6 in, 1 out]
                                }
                                frame #3 {
                                n5496 = local read "Stopper that ends \nthe main loops"() -> (w5898:bool)
                                n5497 = local read "VISA Refnum in\nfor Pump"() -> (w5899:refnum<visa-resource-name>)
                                n5498 = case shown="True" w5898 {
                                frame False {
                                }
                                frame True {
                                n5499 = local read "VISA Refnum in\nfor Pump"() -> (w5900:refnum<visa-resource-name>)
                                n5500 = call "HardStopCurrentProcess (SubVI).vi"("VISA Refnum in"=w5900) -> ()  [unwired: 11 in]
                                }
                                }
                                n5501 = call "ProcessCompletionWaiter (SubVI).vi"("VISA Refnum in"=w5899) -> ()  [unwired: 11 in]
                                }
                                frame #4 {
                                n5502 = local read "VISA Refnum in\nfor Pump"() -> (w5902:refnum<visa-resource-name>)
                                n5503 = call "PortChanger (SubVI).vi"("Port Number"="1", "VISA Refnum in"=w5902) -> ()  [unwired: 10 in]
                                }
                                frame #5 {
                                n5504 = local read "Stopper that ends \nthe main loops"() -> (w5903:bool)
                                n5505 = local read "VISA Refnum in\nfor Pump"() -> (w5904:refnum<visa-resource-name>)
                                n5506 = case shown="True" w5903 {
                                frame False {
                                }
                                frame True {
                                n5507 = local read "VISA Refnum in\nfor Pump"() -> (w5905:refnum<visa-resource-name>)
                                n5508 = call "HardStopCurrentProcess (SubVI).vi"("VISA Refnum in"=w5905) -> ()  [unwired: 11 in]
                                }
                                }
                                n5509 = call "ProcessCompletionWaiter (SubVI).vi"("VISA Refnum in"=w5904) -> ()  [unwired: 11 in]
                                }
                                frame #6 {
                                n5510 = local read "VISA Refnum in\nfor Pump"() -> (w5910:refnum<visa-resource-name>)
                                n5511 = local read "Volume of Syringe"() -> (w5907:dbl)
                                n5512 = call "GoToAbsolutePosition(SubVI).vi"("Absolute Volume Position in Syringe (in ul)"=0.0, "Volume of Syringe"=w5907, "Resolution of Pumping"=T2."Standard Pumping", "Flow Rate (ul/min)"=150.0, "VISA Refnum in"=w5910) -> ()  [unwired: 6 in, 1 out]
                                }
                                frame #7 {
                                n5513 = local read "Stopper that ends \nthe main loops"() -> (w5911:bool)
                                n5514 = local read "VISA Refnum in\nfor Pump"() -> (w5912:refnum<visa-resource-name>)
                                n5515 = case shown="True" w5911 {
                                frame False {
                                }
                                frame True {
                                n5516 = local read "VISA Refnum in\nfor Pump"() -> (w5913:refnum<visa-resource-name>)
                                n5517 = call "HardStopCurrentProcess (SubVI).vi"("VISA Refnum in"=w5913) -> ()  [unwired: 11 in]
                                }
                                }
                                n5518 = call "ProcessCompletionWaiter (SubVI).vi"("VISA Refnum in"=w5912) -> ()  [unwired: 11 in]
                                }
                                }
                              }
                              frame True {
                                n5519 = for {
                                N: 2 -> [_]
                                n5520 = stacked-sequence {
                                frame #0 {
                                n5521 = local read "VISA Refnum in\nfor Pump"() -> (w5916:refnum<visa-resource-name>)
                                n5522 = local read "Port for \nC2-Elution"() -> (w5915:string)
                                n5523 = call "PortChanger (SubVI).vi"("Port Number"=w5915, "VISA Refnum in"=w5916) -> ()  [unwired: 10 in]
                                }
                                frame #1 {
                                n5524 = local read "VISA Refnum in\nfor Pump"() -> (w5917:refnum<visa-resource-name>)
                                n5525 = call "ProcessCompletionWaiter (SubVI).vi"("VISA Refnum in"=w5917) -> ()  [unwired: 11 in]
                                }
                                frame #2 {
                                n5526 = local read "Buffer-C2 Pumping\nResolution"() -> (w5920:T2)
                                n5527 = local read "VISA Refnum in\nfor Pump"() -> (w5922:refnum<visa-resource-name>)
                                n5528 = local read "Apparent Volume\nof Syringe"() -> (w5918:dbl)
                                n5529 = local read "Volume of Syringe"() -> (w5921:dbl)
                                n5530 = call "RPickUp(SubVI).vi"("Volume to be picked up"=w5918, "Volume of Syringe"=w5921, "Resolution of PickUP"=w5920, "PickUp Flow Rate (ul/min)"=150.0, "VISA Refnum in"=w5922) -> ()  [unwired: 6 in, 1 out]
                                }
                                frame #3 {
                                n5531 = local read "Stopper that ends \nthe main loops"() -> (w5923:bool)
                                n5532 = local read "VISA Refnum in\nfor Pump"() -> (w5924:refnum<visa-resource-name>)
                                n5533 = case shown="True" w5923 {
                                frame False {
                                }
                                frame True {
                                n5534 = local read "VISA Refnum in\nfor Pump"() -> (w5925:refnum<visa-resource-name>)
                                n5535 = call "HardStopCurrentProcess (SubVI).vi"("VISA Refnum in"=w5925) -> ()  [unwired: 11 in]
                                }
                                }
                                n5536 = call "ProcessCompletionWaiter (SubVI).vi"("VISA Refnum in"=w5924) -> ()  [unwired: 11 in]
                                }
                                frame #4 {
                                n5537 = local read "VISA Refnum in\nfor Pump"() -> (w5927:refnum<visa-resource-name>)
                                n5538 = call "PortChanger (SubVI).vi"("Port Number"="1", "VISA Refnum in"=w5927) -> ()  [unwired: 10 in]
                                }
                                frame #5 {
                                n5539 = local read "Stopper that ends \nthe main loops"() -> (w5928:bool)
                                n5540 = local read "VISA Refnum in\nfor Pump"() -> (w5929:refnum<visa-resource-name>)
                                n5541 = case shown="True" w5928 {
                                frame False {
                                }
                                frame True {
                                n5542 = local read "VISA Refnum in\nfor Pump"() -> (w5930:refnum<visa-resource-name>)
                                n5543 = call "HardStopCurrentProcess (SubVI).vi"("VISA Refnum in"=w5930) -> ()  [unwired: 11 in]
                                }
                                }
                                n5544 = call "ProcessCompletionWaiter (SubVI).vi"("VISA Refnum in"=w5929) -> ()  [unwired: 11 in]
                                }
                                frame #6 {
